vi "Pockels Cal-Write meas AI to sys config.vi"(8 "error in (no error)":errorcluster) -> (0 "error out":errorcluster)   [LabVIEW 2017]
uses:
  Typedefs/HW config states enum.ctl
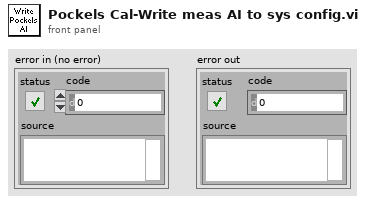
[diagram p1: front panel]
types:
  T1 = typedef "HW config states enum.ctl" = enum16{"Load from file", "Save to file", "Write all", "Read all", "Write XY stage settings", "Write DAQ FPGA settings", "Write Control FPGA settings", "Write Phys Channels", "Clear", "Compare from file"}
  T2 = typedef "Hardware Configuration settings.ctl" = cluster{"Computer MAC address":string, "XY Stage":T3, "Cam VidRec":T4, "Control Sys. HW config":T5, "DAQ FPGA HW Config":cluster{"Target":T6, "input card type":T7}, "DAQmx Chan":T8, "Encoder":T9, "Z Stage config cluster":T10, "Trigger HW config":T11, "Externalise Triggers":bool, "MC Supported":bool, "Laser 1 config cluster":T12, "Prechirper 1 config cluster":T13, "Laser Power Control HW config":T14, "No of AOD":u8, "Dev. PC":bool, "Swap XY on stage":bool, "Axial MC":bool}
  T3 = typedef "XY Stage config cluster.ctl" = cluster{"COM port":refnum<visa-resource-name>, "XY stage available":bool, "Baudrate":i32, "Type":string}
  T4 = typedef "Cam VidRec HW config setup cluster.ctl" = cluster{"DO flag-Video record":tag, "DO flag-Trial start":tag, "VidRec available":bool}
  T5 = typedef "Control Sys HW config cluster.ctl" = cluster{"Control system.FPGA available?":bool, "Control system.FPGA Type":string, "Control system.Network adapter name":string, "Control system.MAC address":string, "Control system.Ethernet Port":u32}
  T6 = typedef "nirio_resource_hc.ctl" = tag
  T7 = typedef "FPGA input type AC-DC.ctl" = enum16{"AC Card", "DC Card"}
  T8 = typedef "DAQmx physical channels cluster.ctl" = cluster{"Pockels AO":tag, "Hard shutter AO":tag, "PMT AOs":tag, "Power meter AI":tag}
  T9 = typedef "Encoder config cluster.ctl" = cluster{"IP address":string, "Port":u16, "Encoder available":bool, "Wheel radius (cm)":dbl, "Encoder Trigger":tag}
  T10 = typedef "Z Stage config cluster.ctl" = cluster{"COM port":refnum<visa-resource-name>, "Z stage available":bool, "Baudrate":i32, "Type":string}
  T11 = typedef "Triggers HW config.ctl" = cluster{"Available Device List":i32, "Device Address":string}
  T12 = typedef "Laser 1 config cluster.ctl" = cluster{"COM port":refnum<visa-resource-name>, "Laser 1 available":bool, "Baud Rate":i32, "Type":string}
  T13 = typedef "PreChirper 1 config cluster.ctl" = cluster{"COM port":refnum<visa-resource-name>, "Prechirper 1 \navailable":bool, "Baud Rate":i32, "Type":string}
  T14 = typedef "Laser Power Control HW config.ctl" = cluster{"Laser Power Control":string, "Laser Power Modulation Control":string}
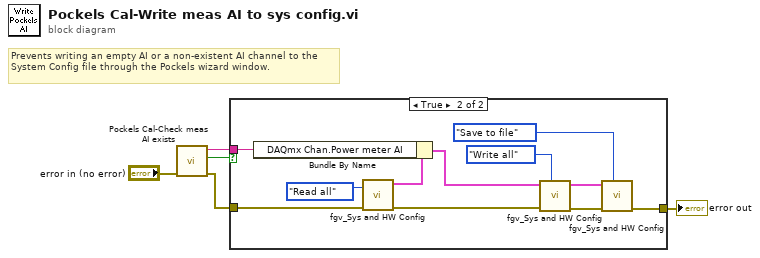
[diagram p0: block diagram]
diagram:
  # "Prevents writing an empty AI or a non-existent AI channel to the System Config file through the Pockels wizard window."
  n1 = call "Pockels Cal-Check meas AI exists.vi"("error in (no error)"="error in (no error)") -> ("error out"=w5:errorcluster, "Power-meter meas. AI channel exists"=w1:bool, "Power meter AI (dupl)"=w2:tag)  [unwired: 8 in]
  n2 = case shown="True" w1 {
    tunnel: w2 -> [_ w11]
    tunnel: w5 -> [w6 w10]
    tunnel: [w6 w9] -> w3
    frame False {
    }
    frame True {
      n3 = call "fgv_Sys and HW Config.vi"("Function"=HW_config_states_enum."Read all", "error in (no error)"=w10) -> ("error out"=w17:errorcluster, "Hardware Configuration OUT"=w14:T2)  [unwired: 7 in, 1 out]
      n4 = Bundle By Name(cluster=w14, "DAQmx Chan.Power meter AI"=w11) -> (w8:T2)
      n5 = call "fgv_Sys and HW Config.vi"("Function"=HW_config_states_enum."Write all", "error in (no error)"=w17, "Hardware Configuration"=w8) -> ("error out"=w16:errorcluster, "Hardware Configuration OUT"=w7:T2)  [unwired: 6 in, 1 out]
      n6 = call "fgv_Sys and HW Config.vi"("Function"=HW_config_states_enum."Save to file", "error in (no error)"=w16, "Hardware Configuration"=w7) -> ("error out"=w9:errorcluster)  [unwired: 6 in, 2 out]
    }
  }
  "error out" <- w3
